vi "AO_mini_DM setup.vi"() -> ()   [LabVIEW 2018]
uses:
  <userlib>/WaveKit.lib/Controls/Wavefront Corrector states - ONE.ctl
  <userlib>/WaveKit.lib/Classes/WavefrontCorrector/WavefrontCorrector.lvclass
  <userlib>/WaveKit.lib/Classes/WavefrontCorrectorSet/WavefrontCorrectorSet.lvclass
  <vilib>/Utility/file.llb/Read From Spreadsheet File (DBL).vi
  <vilib>/Analysis/1siggen.llb/Ramp Pattern by Delta.vi
  <userlib>/WaveKit.lib/Classes/ModalCoef/ModalCoef.lvclass
  <userlib>/WaveKit.lib/Controls/Pupil.lvclass
  <vilib>/Analysis/NI_AALBase.lvlib
panel:
  in  "idxType":enum16{"Wyant", "ANSI"}(ring)
  out "DM Status":sgl[](graph)
  in  "SaveFile":bool
  in  "Output folder":path=path "D:/Data"
  in  "File prefix name":string="Test"
  out "Final Positions":sgl[](array[numeric])
  out "Zern coef out":sgl[](array[numeric])
  out "Zern index out":i32[](array[numeric])
  in  "Update":bool
  in  "Additional file":path=path "D:/SystemAlignment/system_aberration_20191029.dat"
  in  "Input type":T1(ring)=enum."Zernike Coef"
  in  "Additional Command":bool=TRUE
  in  "Initial offset":bool=TRUE
  in  "Haso configuration file":path=path "C:/Program Files (x86)/Imagine Optic/Configuration Files/HASO3_first_7364.dat"
  in  "interaction matrix file":path=path "D:/SystemAlignment/IM_20220706_1p5sx2_0p5um.aomi"
  in  "Initial haso file":path=path "D:/SystemAlignment/system_aberration_residual_20220406.has"
  in  "Zern index in":i32[](array[numeric])
  in  "Zern coef in":sgl[](array[numeric])
  out "error out":errorcluster
  out "Initial Positions":sgl[](array[numeric])
  out "Initial State":T2[](array[typedef])
  out "ActuatorsNumber":i32
  in  "error in (no error)":errorcluster
  in  "Offset command file":path=path "D:/SystemAlignment/system_aberration_20220706.dat"
  in  "DM configuration file":path=path "C:/Program Files (x86)/Imagine Optic/Configuration Files/WaveFrontCorrector_mirao52-e_0326.dat"
  in  "stop":bool
  # "Configuration files"
  # "Commands"
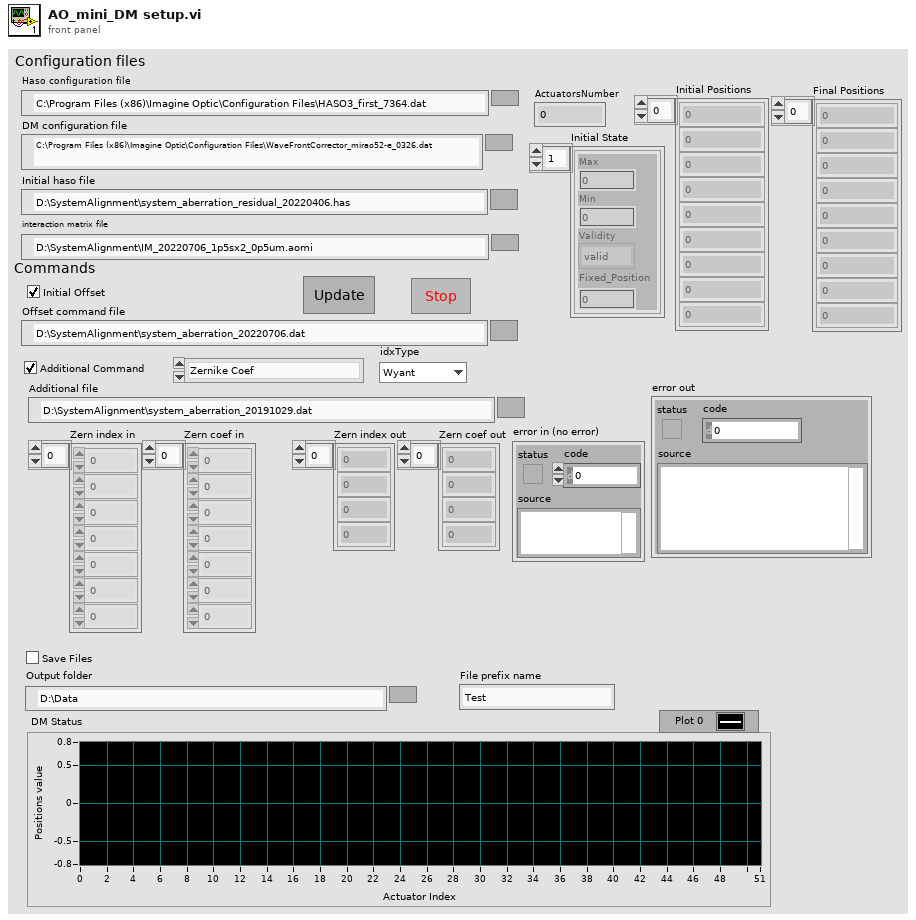
[diagram p1: front panel]
types:
  T1 = enum16{"Zero Input", "Command File", "Zernike Coef", "Zernike File"}
  T2 = typedef "Wavefront Corrector states - ONE.ctl" = cluster{"Max":sgl, "Min":sgl, "Validity":enum16{"valid", "fixed", "invalid"}, "Fixed_Position":sgl}
  T3 = typedef "Wavefront Corrector Position.ctl" = sgl[]
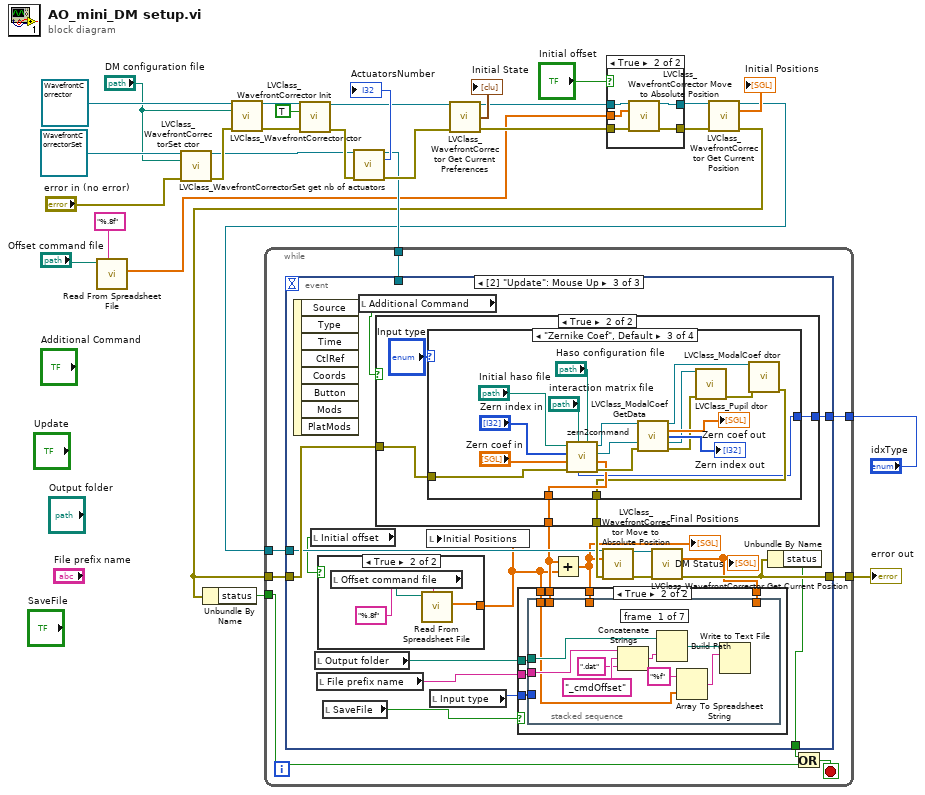
[diagram p0: block diagram]
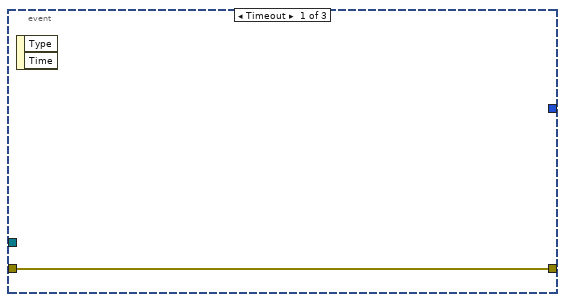
[diagram p3: hidden frame]
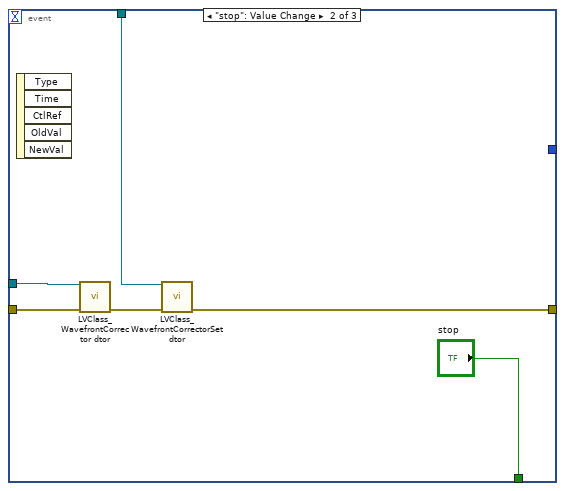
[diagram p4: hidden frame]
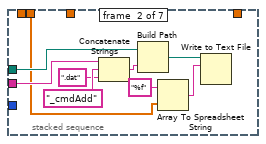
[diagram p6: hidden frame]
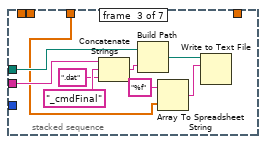
[diagram p7: hidden frame]
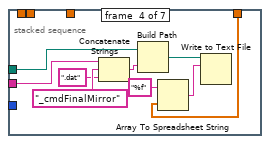
[diagram p8: hidden frame]
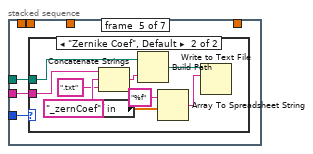
[diagram p9: hidden frame]
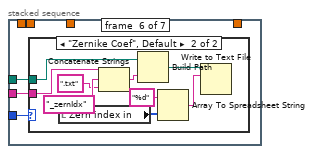
[diagram p11: hidden frame]
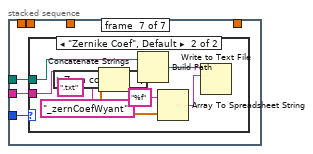
[diagram p13: hidden frame]
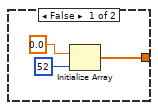
[diagram p15: hidden frame]
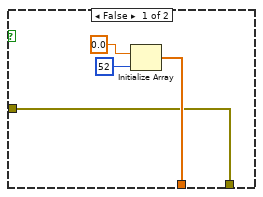
[diagram p16: hidden frame]
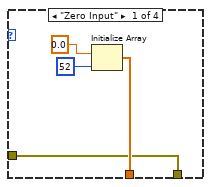
[diagram p17: hidden frame]
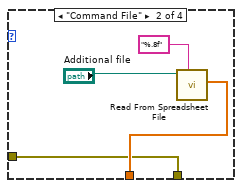
[diagram p18: hidden frame]
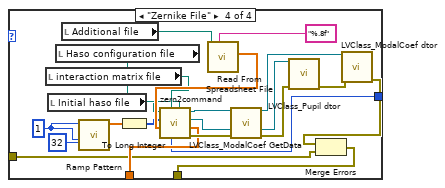
[diagram p19: hidden frame]
diagram:
  n1 = call-poly <vilib>:"Read From Spreadsheet File.vi"("format (%.3f)"="%.8f", "file path (dialog if empty)"="Offset command file") -> ("first row"=w2:dbl[])  [unwired: 5 in, 4 out]
  n2 = call <userlib>:"LVClass_WavefrontCorrectorSet ctor.vi"("WavefrontCorrectorSet in"=refnum<class "WavefrontCorrectorSet.lvclass"> refnum, "PathToWavefrontCorrectorSetupFile"="DM configuration file", "error in (no error)"="error in (no error)") -> ("WavefrontCorrectorSet out"=w16:refnum<class "WavefrontCorrectorSet.lvclass">, "error out"=w25:errorcluster)  [unwired: 11 in]
  n3 = call <userlib>:"LVClass_WavefrontCorrector ctor.vi"("WavefrontCorrector in"=refnum<class "WavefrontCorrector.lvclass"> refnum, "PathToWavefrontCorrectorSetupFile"="DM configuration file", "error in (no error)"=w25) -> ("WavefrontCorrector out"=w20:refnum<class "WavefrontCorrector.lvclass">, "error out"=w19:errorcluster)  [unwired: 11 in]
  n4 = call <userlib>:"LVClass_WavefrontCorrector Init.vi"("WavefrontCorrector in"=w20, "set_init_state_from_config_file"=TRUE, "error in (no error)"=w19) -> ("WavefrontCorrector out"=w14:refnum<class "WavefrontCorrector.lvclass">, "error out"=w18:errorcluster)  [unwired: 11 in]
  n5 = call <userlib>:"LVClass_WavefrontCorrectorSet get nb of actuators.vi"("WavefrontCorrectorSet in"=w16, "error in (no error)"=w18) -> ("WavefrontCorrectorSet out"=w9:refnum<class "WavefrontCorrectorSet.lvclass">, "ActuatorsNumber"=→"ActuatorsNumber":i32, "error out"=w15:errorcluster)  [unwired: 11 in]
  n6 = call <userlib>:"LVClass_WavefrontCorrector Get Current Preferences.vi"("WavefrontCorrector in"=w14, "error in (no error)"=w15) -> ("WavefrontCorrector out"=w6:refnum<class "WavefrontCorrector.lvclass">, "Mirror preferences.Wavefront Corrector State"=→"Initial State":T2[], "error out"=w5:errorcluster)  [unwired: 10 in, 1 out]
  n7 = case shown="True" "Initial offset" {
    tunnel: w2 -> [_ w36]
    tunnel: [w31 w35] -> w11
    tunnel: [w30 w34] -> w10
    tunnel: w6 -> [w31 w33]
    tunnel: w5 -> [w30 w32]
    frame False {
    }
    frame True {
      n8 = call <userlib>:"LVClass_WavefrontCorrector Move to Absolute Position.vi"("WavefrontCorrector in"=w33, "Absolute Positions"=w36, "error in (no error)"=w32) -> ("WavefrontCorrector out"=w35:refnum<class "WavefrontCorrector.lvclass">, "error out"=w34:errorcluster)  [unwired: 11 in]
    }
  }
  n9 = call <userlib>:"LVClass_WavefrontCorrector Get Current Position.vi"("WavefrontCorrector in"=w11, "error in (no error)"=w10) -> ("WavefrontCorrector out"=w3:refnum<class "WavefrontCorrector.lvclass">, "Wavefront Corrector Position"=→"Initial Positions":T3, "error out"=w8:errorcluster)  [unwired: 11 in]
  n10 = Unbundle By Name(w8) -> ("status"=w28:bool)
  n11 = while {
    tunnel: w28 -> [w43]
    tunnel: w9 -> [w41]
    tunnel: w3 -> [w40]
    tunnel: w8 -> [w39]
    tunnel: [w38] -> w7
    tunnel: "idxType" -> [w37]
    stop <- w42 stop-if-true
    n12 = event shown="[2] \"Update\": Mouse Up" {
      selector: _ -> [_ _ _]
      dyn-events: _ -> [_ _ _]
      timeout: _ -> [_ _ _]
      tunnel: [_ "stop" w66] -> w44
      tunnel: w41 -> [_ w50 _]
      tunnel: w40 -> [_ w49 w62]
      tunnel: w39 -> [w45 w48 w69]
      tunnel: [w45 w46 w67] -> w38
      tunnel: w37 -> [_ _ w52]
      event Timeout {
        n13 = event-data() -> ()  [unwired: 1 in, 2 out]
      }
      event "stop": Value Change {
        n14 = event-data() -> ()  [unwired: 1 in, 5 out]
        n15 = call <userlib>:"LVClass_WavefrontCorrector dtor.vi"("WavefrontCorrector in"=w49, "error in (no error)"=w48) -> ("error out"=w47:errorcluster)  [unwired: 12 in, 1 out]
        n16 = call <userlib>:"LVClass_WavefrontCorrectorSet dtor.vi"("WavefrontCorrectorSet in"=w50, "error in (no error)"=w47) -> ("error out"=w46:errorcluster)  [unwired: 12 in, 1 out]
      }
      event "Update": Mouse Up {
        n17 = event-data() -> ()  [unwired: 1 in, 8 out]
        n18 = local read "Initial offset"() -> (w61:bool)
        n19 = local read "Output folder"() -> (w59:path)
        n20 = local read "File prefix name"() -> (w58:string)
        n21 = case shown="True" w61 {
          tunnel: [w149 w154] -> w54
          frame False {
            n22 = Initialize Array(0.0, 52) -> (w149:dbl[])
          }
          frame True {
            n23 = local read "Offset command file"() -> (w153:path)
            n24 = call-poly <vilib>:"Read From Spreadsheet File.vi"("format (%.3f)"="%.8f", "file path (dialog if empty)"=w153) -> ("first row"=w154:dbl[])  [unwired: 5 in, 4 out]
          }
        }
        n25 = local read "SaveFile"() -> (w60:bool)
        n26 = local read "Additional Command"() -> (w68:bool)
        n27 = case shown="True" w68 {
          tunnel: w69 -> [w155 w163]
          tunnel: [w156 w161] -> w57
          tunnel: [w155 w160] -> w63
          tunnel: w52 -> [_ w159]
          frame False {
            n28 = Initialize Array(0.0, 52) -> (w156:dbl[])
          }
          frame True {
            n29 = case shown="\"Zernike Coef\", Default" "Input type" {
              tunnel: w163 -> [w164 w168 w176 w192]
              tunnel: [w165 w169 w174 w194] -> w161
              tunnel: [w164 w168 w173 w191] -> w160
              tunnel: w159 -> [_ _ w172 w190]
              frame "Zero Input" {
                n30 = Initialize Array(0.0, 52) -> (w165:dbl[])
              }
              frame "Command File" {
                n31 = call-poly <vilib>:"Read From Spreadsheet File.vi"("format (%.3f)"="%.8f", "file path (dialog if empty)"="Additional file") -> ("first row"=w169:dbl[])  [unwired: 5 in, 4 out]
              }
              frame "Zernike Coef", Default {
                n32 = call "zern2command.vi"("Haso configuration file"="Haso configuration file", "idxType"=w172, "interaction matrix file"="interaction matrix file", "error in (no error)"=w176, "Zern coef in"="Zern coef in", "Zern index in"="Zern index in", "Initial haso file"="Initial haso file") -> ("error out"=w175:errorcluster, "Offset Positions"=w174:sgl[], "Zern pupil out"=w177:refnum<class "Pupil.lvclass">, "ModalCoef out"=w178:refnum<class "ModalCoef.lvclass">)  [unwired: 1 in]
                n33 = call <userlib>:"LVClass_ModalCoef GetData.vi"("ModalCoef in"=w178, "Pupil.lvclass"=w177, "error in (no error)"=w175) -> ("ModalCoef out"=w184:refnum<class "ModalCoef.lvclass">, "coef"=→"Zern coef out":sgl[], "index"=→"Zern index out":u32[], "Pupil.lvclass (dup)"=w181:refnum<class "Pupil.lvclass">, "error out"=w180:errorcluster)  [unwired: 8 in]
                n34 = call <userlib>:"LVClass_Pupil dtor.vi"("Pupil in"=w181, "error in (no error)"=w180) -> ("error out"=w179:errorcluster)  [unwired: 12 in, 1 out]
                n35 = call <userlib>:"LVClass_ModalCoef dtor.vi"("ModalCoef in"=w184, "error in (no error)"=w179) -> ("error out"=w173:errorcluster)  [unwired: 12 in, 1 out]
              }
              frame "Zernike File" {
                w197 = 1
                n36 = local read "interaction matrix file"() -> (w201:path)
                n37 = local read "Initial haso file"() -> (w199:path)
                n38 = local read "Haso configuration file"() -> (w200:path)
                n39 = local read "Additional file"() -> (w210:path)
                n40 = call-poly <vilib>:"Ramp Pattern.vi"("start"=w197, "end"=32, "delta"=w197) -> ("Ramp Pattern"=w198:dbl[])  [unwired: 6 in, 2 out]
                n41 = To Long Integer(number=w198) -> (32bit integer=w195:i32[])
                n42 = call-poly <vilib>:"Read From Spreadsheet File.vi"("format (%.3f)"="%.8f", "file path (dialog if empty)"=w210) -> ("first row"=w202:dbl[])  [unwired: 5 in, 4 out]
                n43 = call "zern2command.vi"("Haso configuration file"=w200, "idxType"=w190, "interaction matrix file"=w201, "Zern coef in"=w202, "Zern index in"=w195, "Initial haso file"=w199) -> ("error out"=w203:errorcluster, "Offset Positions"=w194:sgl[], "Zern pupil out"=w204:refnum<class "Pupil.lvclass">, "ModalCoef out"=w205:refnum<class "ModalCoef.lvclass">)  [unwired: 2 in]
                n44 = call <userlib>:"LVClass_ModalCoef GetData.vi"("ModalCoef in"=w205, "Pupil.lvclass"=w204, "error in (no error)"=w203) -> ("ModalCoef out"=w209:refnum<class "ModalCoef.lvclass">, "Pupil.lvclass (dup)"=w208:refnum<class "Pupil.lvclass">, "error out"=w207:errorcluster)  [unwired: 8 in, 2 out]
                n45 = call <userlib>:"LVClass_Pupil dtor.vi"("Pupil in"=w208, "error in (no error)"=w207) -> ("error out"=w206:errorcluster)  [unwired: 12 in, 1 out]
                n46 = call <userlib>:"LVClass_ModalCoef dtor.vi"("ModalCoef in"=w209, "error in (no error)"=w206) -> ("error out"=w193:errorcluster)  [unwired: 12 in, 1 out]
                n47 = Merge Errors(w193, w192) -> (w191:errorcluster)
              }
            }
          }
        }
        n48 = local write "Initial Positions"(w54) -> ()
        n49 = local read "Input type"() -> (w56:T1)
        n50 = Add(x=w57, y=w54) -> (x+y=w55:dbl[])
        "Final Positions" <- w55
        n51 = call <userlib>:"LVClass_WavefrontCorrector Move to Absolute Position.vi"("WavefrontCorrector in"=w62, "Absolute Positions"=w55, "error in (no error)"=w63) -> ("WavefrontCorrector out"=w64:refnum<class "WavefrontCorrector.lvclass">, "error out"=w65:errorcluster)  [unwired: 11 in]
        n52 = call <userlib>:"LVClass_WavefrontCorrector Get Current Position.vi"("WavefrontCorrector in"=w64, "error in (no error)"=w65) -> ("Wavefront Corrector Position"=w53:T3, "error out"=w67:errorcluster)  [unwired: 11 in, 1 out]
        "DM Status" <- w53
        n53 = case shown="True" w60 {
          tunnel: w59 -> [_ w76]
          tunnel: w58 -> [_ w75]
          tunnel: w54 -> [_ w74]
          tunnel: w57 -> [_ w73]
          tunnel: w55 -> [_ w72]
          tunnel: w56 -> [_ w71]
          tunnel: w53 -> [_ w70]
          frame False {
          }
          frame True {
            n54 = stacked-sequence {
              tunnel: w76 -> [w81 w90 w99 w108 w115 w127 w139]
              tunnel: w75 -> [w79 w88 w97 w106 w114 w126 w138]
              tunnel: w74 -> [w77 _ _ _ _ _ _]
              tunnel: w73 -> [_ w86 _ _ _ _ _]
              tunnel: w72 -> [_ _ w95 _ _ _ _]
              tunnel: w71 -> [_ _ _ _ w113 w125 w137]
              tunnel: w70 -> [_ _ _ w104 _ _ _]
              frame #0 {
                n55 = Concatenate Strings(w79, "_cmdOffset", ".dat") -> (w82:string)
                n56 = Build Path(base path=w81, name or relative path=w82) -> (appended path=w83:path)
                n57 = Array To Spreadsheet String(array=w77, 3:"%f") -> (spreadsheet string=w84:string)  [unwired: 1 in]
                n58 = Write to Text File(file (use dialog)=w83, text=w84) -> ()  [unwired: 2 in, 3 out]
              }
              frame #1 {
                n59 = Concatenate Strings(w88, "_cmdAdd", ".dat") -> (w91:string)
                n60 = Build Path(base path=w90, name or relative path=w91) -> (appended path=w92:path)
                n61 = Array To Spreadsheet String(array=w86, 3:"%f") -> (spreadsheet string=w93:string)  [unwired: 1 in]
                n62 = Write to Text File(file (use dialog)=w92, text=w93) -> ()  [unwired: 2 in, 3 out]
              }
              frame #2 {
                n63 = Concatenate Strings(w97, "_cmdFinal", ".dat") -> (w100:string)
                n64 = Build Path(base path=w99, name or relative path=w100) -> (appended path=w101:path)
                n65 = Array To Spreadsheet String(array=w95, 3:"%f") -> (spreadsheet string=w102:string)  [unwired: 1 in]
                n66 = Write to Text File(file (use dialog)=w101, text=w102) -> ()  [unwired: 2 in, 3 out]
              }
              frame #3 {
                n67 = Concatenate Strings(w106, "_cmdFinalMirror", ".dat") -> (w109:string)
                n68 = Build Path(base path=w108, name or relative path=w109) -> (appended path=w110:path)
                n69 = Array To Spreadsheet String(array=w104, 3:"%f") -> (spreadsheet string=w111:string)  [unwired: 1 in]
                n70 = Write to Text File(file (use dialog)=w110, text=w111) -> ()  [unwired: 2 in, 3 out]
              }
              frame #4 {
                n71 = case shown="\"Zernike Coef\", Default" w113 {
                  tunnel: w115 -> [_ w120]
                  tunnel: w114 -> [_ w118]
                  frame "Zero Input" {
                  }
                  frame "Zernike Coef", Default {
                    n72 = local read "Zern coef in"() -> (w116:sgl[])
                    n73 = Concatenate Strings(w118, "_zernCoef", ".txt") -> (w121:string)
                    n74 = Build Path(base path=w120, name or relative path=w121) -> (appended path=w122:path)
                    n75 = Array To Spreadsheet String(array=w116, 3:"%f") -> (spreadsheet string=w123:string)  [unwired: 1 in]
                    n76 = Write to Text File(file (use dialog)=w122, text=w123) -> ()  [unwired: 2 in, 3 out]
                  }
                }
              }
              frame #5 {
                n77 = case shown="\"Zernike Coef\", Default" w125 {
                  tunnel: w127 -> [_ w132]
                  tunnel: w126 -> [_ w130]
                  frame "Zero Input" {
                  }
                  frame "Zernike Coef", Default {
                    n78 = local read "Zern index in"() -> (w128:i32[])
                    n79 = Concatenate Strings(w130, "_zernIdx", ".txt") -> (w133:string)
                    n80 = Build Path(base path=w132, name or relative path=w133) -> (appended path=w134:path)
                    n81 = Array To Spreadsheet String(array=w128, 3:"%d") -> (spreadsheet string=w135:string)  [unwired: 1 in]
                    n82 = Write to Text File(file (use dialog)=w134, text=w135) -> ()  [unwired: 2 in, 3 out]
                  }
                }
              }
              frame #6 {
                n83 = case shown="\"Zernike Coef\", Default" w137 {
                  tunnel: w139 -> [_ w144]
                  tunnel: w138 -> [_ w142]
                  frame "Zero Input" {
                  }
                  frame "Zernike Coef", Default {
                    n84 = local read "Zern coef out"() -> (w140:sgl[])
                    n85 = Concatenate Strings(w142, "_zernCoefWyant", ".txt") -> (w145:string)
                    n86 = Build Path(base path=w144, name or relative path=w145) -> (appended path=w146:path)
                    n87 = Array To Spreadsheet String(array=w140, 3:"%f") -> (spreadsheet string=w147:string)  [unwired: 1 in]
                    n88 = Write to Text File(file (use dialog)=w146, text=w147) -> ()  [unwired: 2 in, 3 out]
                  }
                }
              }
            }
          }
        }
        n89 = Unbundle By Name(w67) -> ("status"=w66:bool)
      }
    }
    n90 = Or(x=w44, y=w43) -> (x .or. y?=w42:bool)
  }
  "error out" <- w7
